vi "readHdfAndAttributes.vi"(11 "HDF5 Path or Ref":path=path "C:/Users/Lino P/Documents/000 - USFQ/TesisDev/data/daq_test/synth_test.h5") -> (1 "Attribute Name(s) out":string[](array[string]), 5 "Data out":dbl[][](array[numeric]))   [LabVIEW 2017]
uses:
  <vilib>/Utility/miscctls.llb/LVRectTypeDef.ctl
  <vilib>/UPVI/lvhdf5/group.llb/H5G_obj_t.ctl
  <vilib>/UPVI/lvhdf5/file.llb/LVH5F Operation.ctl
  <vilib>/UPVI/lvhdf5/dataset.llb/LVH5D Operation.ctl
  <vilib>/UPVI/lvhdf5/identifier.llb/Not an HDF5 Refnum Constant.vi
  <vilib>/UPVI/lvhdf5/common.llb/To HDF5 Ref.vi
  <vilib>/UPVI/lvhdf5/file.llb/H5Fopen.vi
  <vilib>/UPVI/lvhdf5/utility.llb/Select HDF5 Dialog.vi
  <vilib>/UPVI/lvhdf5/utility.llb/Select HDF5 Dialog (File and Object).vi
  <vilib>/UPVI/lvhdf5/dataset.llb/Simple H5Dread (Variant).vi
  <vilib>/UPVI/lvhdf5/attribute.llb/Read Multiple Attributes (Variant).vi
  <vilib>/UPVI/lvhdf5/dataset.llb/H5Dclose.vi
  <vilib>/UPVI/lvhdf5/file.llb/H5Fclose.vi
  <vilib>/UPVI/lvhdf5/dataset.llb/Read Dataset and All Attributes.xnode
  <vilib>/UPVI/lvhdf5/library.llb/HDF5 Ref.ctl
  <vilib>/UPVI/lvhdf5/utility.llb/Select HDF5 Dialog (Object Only).vi
  <vilib>/UPVI/lvhdf5/dataset.llb/OpenCreateReplace Dataset.vi
  <vilib>/UPVI/lvhdf5/dataset.llb/H5Dget_space.vi
  <vilib>/UPVI/lvhdf5/dataspace.llb/H5Sget_simple_extent_dims.vi
  <vilib>/UPVI/lvhdf5/dataspace.llb/H5Sselect_hyperslab.vi
  <vilib>/UPVI/lvhdf5/dataset.llb/H5Dread (Variant).vi
  <vilib>/UPVI/lvhdf5/attribute.llb/private/LVH5AreadWDTAttrs.vi
  <vilib>/UPVI/lvhdf5/dataspace.llb/H5Sclose.vi
  <vilib>/Utility/error.llb/Error Cluster From Error Code.vi
  <vilib>/Utility/VariantDataType/GetClusterInfo.vi
  <vilib>/Utility/VariantDataType/VariantType.lvlib
  <vilib>/Utility/VariantDataType/GetTypeInfo.vi
  <vilib>/UPVI/lvhdf5/attribute.llb/Attribute Array to Cluster.xnode
panel:
  out "z_distance":dbl
  out "sample_freq":dbl
  out "sample_time":dbl
  out "first array":dbl[](array[numeric])
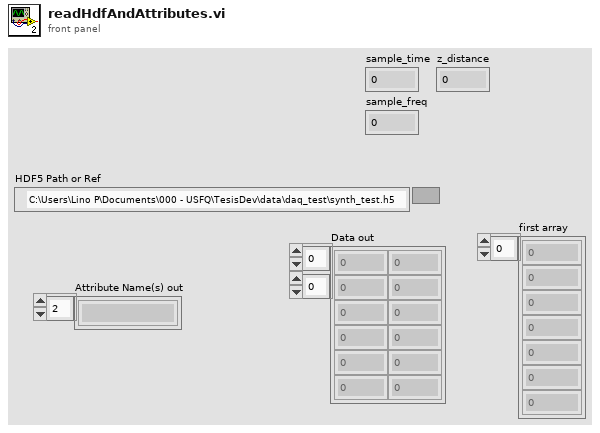
[diagram p1: front panel]
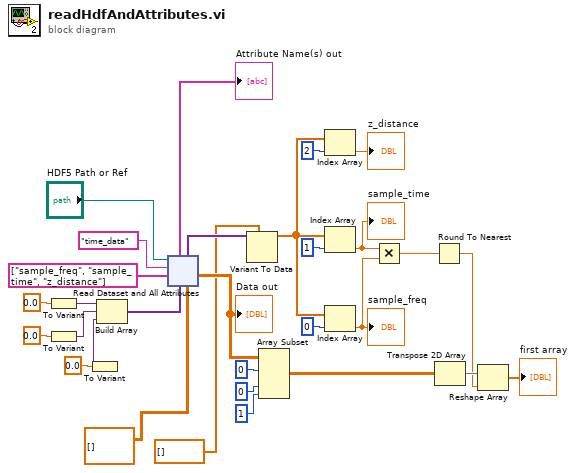
[diagram p0: block diagram]
diagram:
  n1 = To Variant(anything=0.0) -> (Variant=w12:variant)
  n2 = To Variant(anything=0.0) -> (Variant=w13:variant)
  n3 = To Variant(anything=0.0) -> (Variant=w1:variant)
  n4 = Build Array(w12, w13, w1) -> (w11:variant[])
  n5 = xnode "Read Dataset and All Attributes"("Dataset Path"="time_data", "HDF5 Path or Ref"="HDF5 Path or Ref", "Attribute Name(s)"=string[] ["sample_freq", "sample_time", "z_distance"], "Attribute Value(s)"=w11, "Data"=dbl[][] [] ("Array in")) -> ("Attribute Name(s) out"=→"Attribute Name(s) out":string[], "Attribute Value(s) out"=w10:variant[], "Data out"=w29:dbl[][])  [unwired: 1 in, 3 out]
  "Data out" <- w29
  n6 = Variant To Data(type=dbl[] [] ("Array in"), Variant=w10) -> (data=w4:dbl[])  [unwired: 1 in, 1 out]
  n7 = Array Subset(array=w29, index (row)=0 ("index"), index (col)=0 ("index"), length (col)=1 ("length")) -> (w17:dbl[][])  [unwired: 1 in]
  n8 = Index Array(array=w4, index=2) -> (element=→"z_distance":dbl)
  n9 = Index Array(array=w4, index=1) -> (element=w26:dbl)
  "sample_time" <- w26
  n10 = Index Array(array=w4, index=0) -> (element=w27:dbl)
  "sample_freq" <- w27
  n11 = Multiply(x=w26, y=w27) -> (x*y=w6:dbl)
  n12 = Round To Nearest(number=w6) -> (nearest integer value=w5:dbl)
  n13 = Transpose 2D Array(2D array=w17) -> (transposed array=w16:dbl[][])
  n14 = Reshape Array(w16, w5) -> (→"first array":dbl[])
